vi "realWorldToNativeUnits.vi"(9 "velocity (ft/s)":dbl, 11 "position (ft)":dbl) -> (1 "velocity (u/100ms)":dbl, 3 "position (u)":dbl)   [LabVIEW 2017]
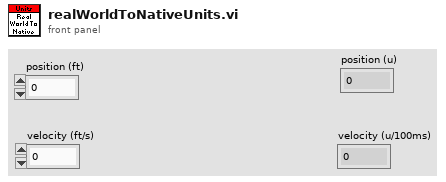
[diagram p1: front panel]
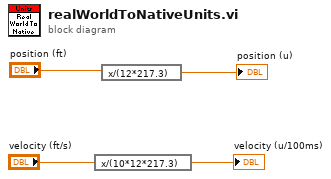
[diagram p0: block diagram]
diagram:
  n1 = expression code="x/(10*12*217.3)"("velocity (ft/s)") -> (→"velocity (u/100ms)":dbl)
  n2 = expression code="x/(12*217.3)"("position (ft)") -> (→"position (u)":dbl)
